vi "INI Initial Value Functional Variable_DStr-Scope SP.vi"(7 "Mode(Get)":T2=enum."Get", 9 "error in":errorcluster caption="Error in", 10 "Value in":T1) -> (1 "error out":errorcluster caption="Error out", 2 "Value out":T1)   [LabVIEW 2012]
uses:
  Function Variable Parameter Operations-Scope SP.ctl
  INI Initial Values_DStr-Scope SP.ctl
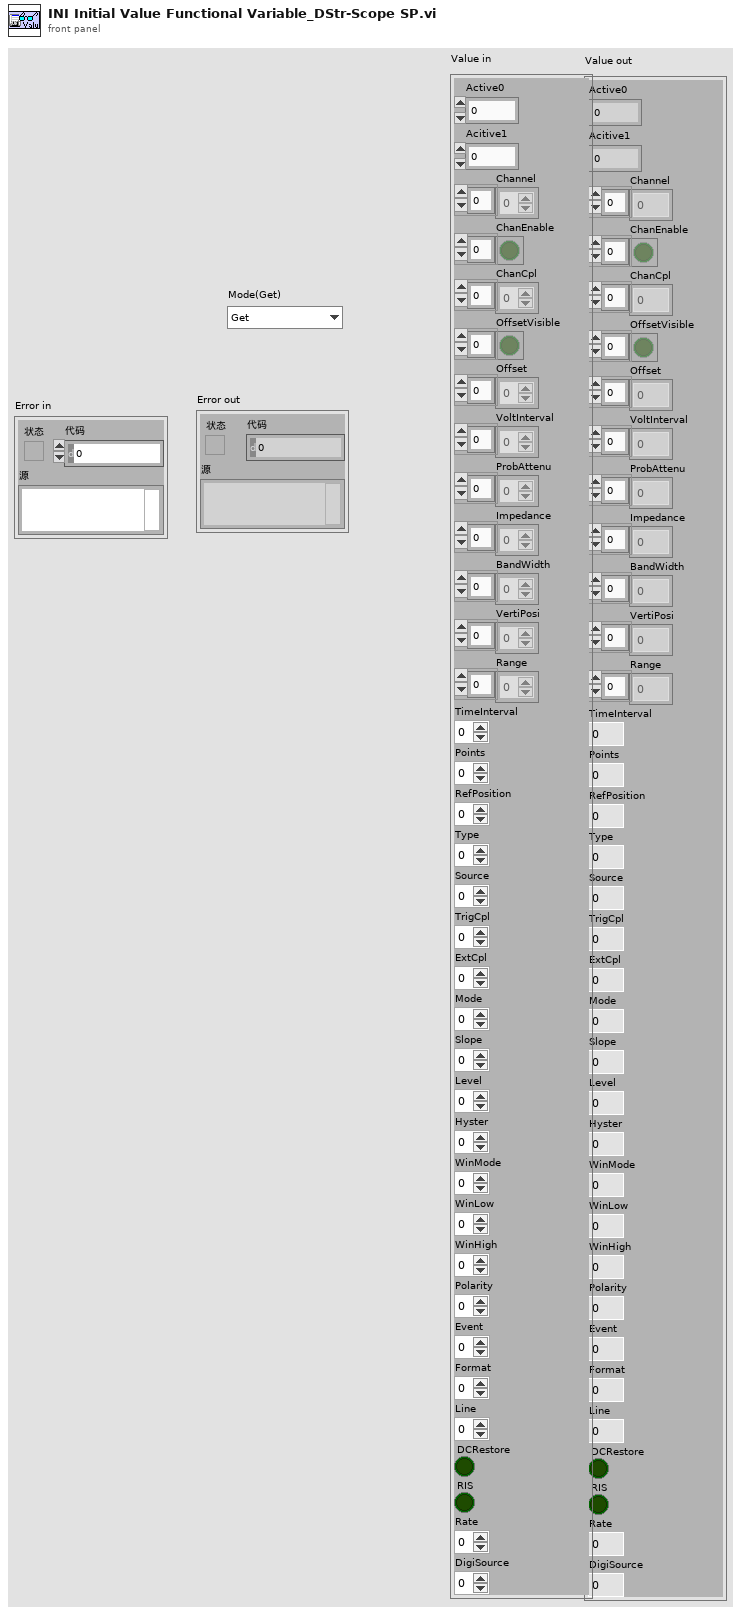
[diagram p1: front panel]
types:
  T1 = typedef "INI Initial Values_DStr-Scope SP.ctl" = cluster{"Active0":i32, "Acitive1":i32, "Channel":i32[], "ChanEnable":bool[], "ChanCpl":i32[], "OffsetVisible":bool[], "Offset":dbl[], "VoltInterval":i32[], "ProbAttenu":i32[], "Impedance":i32[], "BandWidth":i32[], "VertiPosi":dbl[], "Range":dbl[], "TimeInterval":i32, "Points":i32, "RefPosition":dbl, "Type":i32, "Source":i32, "TrigCpl":i32, "ExtCpl":i32, "Mode":i32, "Slope":i32, "Level":dbl, "Hyster":dbl, "WinMode":i32, "WinLow":dbl, "WinHigh":dbl, "Polarity":i32, "Event":i32, "Format":i32, "Line":i32, "DCRestore":bool, "RIS":bool, "Rate":dbl, "DigiSource":i32}
  T2 = typedef "Function Variable Parameter Operations-Scope SP.ctl" = enum16{"Set", "Get"}
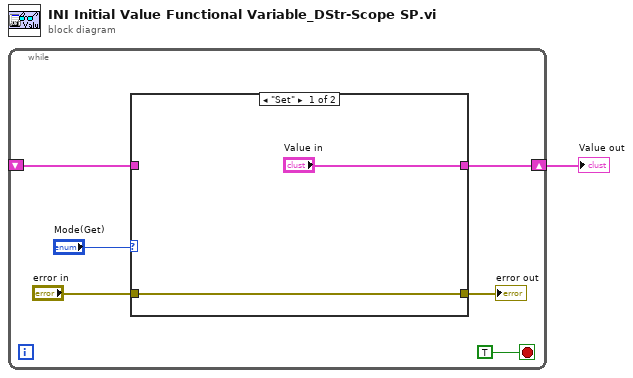
[diagram p0: block diagram]
diagram:
  n1 = while {
    shift-right: [w5] -> w1
    shift-left: _ -> [w4]
    stop <- TRUE stop-if-true
    n2 = case shown="\"Set\"" "Mode(Get)" {
      tunnel: ["Value in" w11] -> w5
      tunnel: w4 -> [_ w11]
      tunnel: [w8 w10] -> w3
      tunnel: "error in" -> [w8 w10]
      frame "Set" {
      }
      frame "Get", Default {
      }
    }
    "error out" <- w3
  }
  "Value out" <- w1
